vi "Update Color Pair Array.vi"(8 "error in (no error)":errorcluster, 9 "Color Pair Array":cluster{"Color":u32, "String":string}[](array[cluster]), 11 "3D Pie.lvclass in":refnum<class "3D Pie.lvclass">) -> (0 "error out":errorcluster, 3 "3D Pie.lvclass out":refnum<class "3D Pie.lvclass">)   [LabVIEW 2020, in "3D Pie.lvclass"]
uses:
  <vilib>/Math Plots/3D Math Plots/3D Pie/3D Pie/3D Pie.lvclass
  e:/builds/penguin/labview/branches/2020/dev/dist/vi.lib/Math Plots/3D Math Plots/3D Plot/3D Plot/3D Plot.lvclass
  <vilib>/Math Plots/3D Math Plots/3D Pie/3D Pie/3D Pie.lvclass/3D Pie.ctl
  <vilib>/Math Plots/3D Math Plots/3D Plot/3D Plot/3D Plot.lvclass
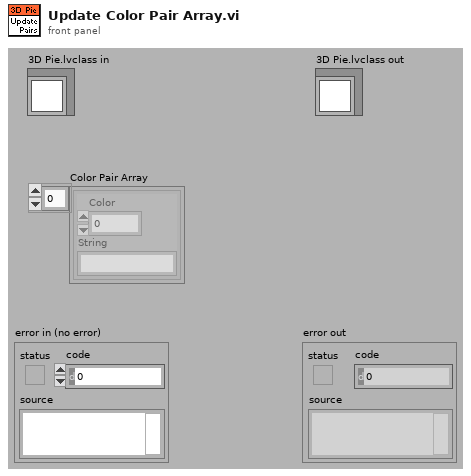
[diagram p1: front panel]
types:
  T1 = typedef "3D Pie.lvclass/3D Pie Property Array.ctl" = T2[]
  T2 = typedef "3D Pie.lvclass/3D Pie Property.ctl" = cluster{"General Property":cluster{"Plot Name":string, "Coordinate System":enum16{"Cartesian", "Cylindrical", "Spherical"}, "Opacity":sgl}, "Projection Property":cluster{"Draw XY":bool, "Draw YZ":bool, "Draw XZ":bool}, "Plot Property":cluster{"Line Style":T3, "Line Width":sgl, "Line Color":u32, "Antialiasing":bool}, "Pie Property":cluster{"Pie Height":sgl, "Pie Center":cluster{"X":sgl, "Y":sgl, "Z":sgl}, "Label Mode":enum16{"None", "Show Percentage", "Show String"}, "Label Size":u16, "Label Color":u32, "Color Pair Array":cluster{"Color":u32, "String":string}[], "Slice Offset?":bool}}
  T3 = typedef "3D Plot.lvclass/Line Type.ctl" = enum16{"None", "Solid", "Dash", "Dot", "Dash Dot"}
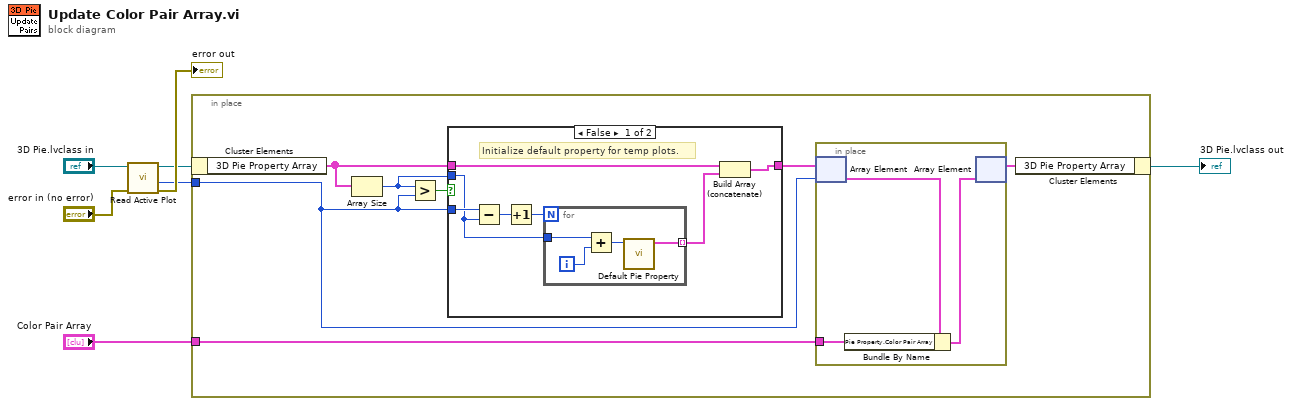
[diagram p0: block diagram]
diagram:
  n1 = call <vilib>:"Read Active Plot.vi"("error in (no error)"="error in (no error)", "3D Plot.lvclass in"="3D Pie.lvclass in") -> ("error out"=→"error out":errorcluster, "Active Plot"=w1:i32, "3D Plot.lvclass out"=w2:refnum<class "3D Pie.lvclass">)  [unwired: 7 out]
  n2 = in-place {
    in-place-border: w1 -> [w9]
    in-place-border: "Color Pair Array" -> [w14]
    n3 = in-place-cluster #1(w2) -> ("3D Pie Property Array"=w12:T1)
    n4 = Array Size(array=w12) -> (size(s)=w8:i32)
    n5 = Greater?(x=w8, y=w9) -> (0:w10:bool)
    n6 = case shown="False" w10 {
      tunnel: [w19 w26] -> w11
      tunnel: w12 -> [w21 w26]
      tunnel: w8 -> [w15 _]
      tunnel: w9 -> [w16 _]
      frame False {
        # "Initialize default property for temp plots."
        n7 = Subtract(x=w16, y=w15) -> (x-y=w18:i32)
        n8 = Increment(x=w18) -> (x+1=w17:i32)
        n9 = for {
          N: w17 -> [_]
          tunnel: w15 -> [w24]
          tunnel: [w22] -> w20 mode=indexing
          i -> [w25]
          n10 = Add(x=w24, y=w25) -> (x+y=w23:i32)
          n11 = call <vilib>:"Default Pie Property.vi"("Plot ID"=w23) -> ("Default Property"=w22:T2)  [unwired: 10 out]
        }
        n12 = Build Array (concatenate)(w21, w20) -> (w19:T1)
      }
      frame True {
      }
    }
    n13 = in-place {
      in-place-border: w14 -> [w27]
      n14 = in-place-array #2(w11, w9) -> (w28:T2)
      n15 = Bundle By Name(cluster=w28, "Pie Property.Color Pair Array"=w27) -> (w29:T2)
      n16 = in-place-array #2(w29) -> (w13:T1)  [unwired: 1 out]
    }
    n17 = in-place-cluster #1("3D Pie Property Array"=w13) -> (→"3D Pie.lvclass out":refnum<class "3D Pie.lvclass">)
  }
